vi "Suite.vi"(8 "error in (no error)":errorcluster, 11 "Global Fixture Test Case Class in":refnum<class "Global Fixture Test Case.lvclass">) -> (0 "error out":errorcluster, 2 "LUnit Test Suite Out":refnum<class "Test Suite.lvclass">, 3 "LUnit Global Fixture Test Case out":refnum<class "Global Fixture Test Case.lvclass">)   [LabVIEW 2020, in "Global Fixture Test Case.lvclass"]
uses:
  Global Fixture Test Case.lvclass
  <vilib>/Astemes/LUnit/Test Suite.lvclass
  Test Suite with Global Fixture/Test Suite with Global Fixture.lvclass
  C:/Program Files (x86)/National Instruments/LabVIEW 2020/vi.lib/Astemes/LUnit/Test Suite.lvclass
  <vilib>/Astemes/LUnit/Test Case.lvclass
  Global Fixture Test Case.lvclass/Global Fixture Test Case.ctl
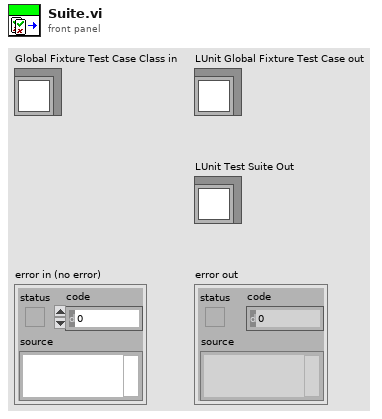
[diagram p1: front panel]
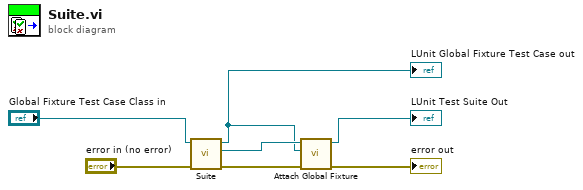
[diagram p0: block diagram]
diagram:
  n1 = call-parent "Suite.vi"("error in (no error)"="error in (no error)", "Test Case Class in"="Global Fixture Test Case Class in") -> ("error out"=w7:errorcluster, "LUnit Test Suite Out"=w3:refnum<class "Test Suite.lvclass">, "LUnit Test Case out"=w1:refnum<class "Global Fixture Test Case.lvclass">)  [unwired: 7 in]
  "LUnit Global Fixture Test Case out" <- w1
  n2 = call "Attach Global Fixture.vi"("error in (no error)"=w7, "Global Fixture Test Case"=w1, "Test Suite.lvclass"=w3) -> ("error out"=→"error out":errorcluster, "Test Suite with Global Fixture"=→"LUnit Test Suite Out":refnum<class "Test Suite with Global Fixture.lvclass">)  [unwired: 7 in]
